vi "Get Range.vi"(11 "Exponential Fit in":refnum<class "Exponential Fit.lvclass">) -> (0 "Ymax":dbl, 1 "Ymin":dbl, 2 "Y Range":dbl, 3 "Exponential Fit out":refnum<class "Exponential Fit.lvclass">)   [LabVIEW 2013, in "Exponential Fit.lvclass"]
uses:
  Exponential Fit.lvclass
  Exponential Fit.lvclass/Exponential Fit.ctl
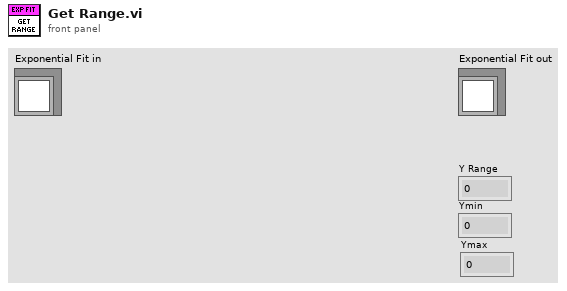
[diagram p1: front panel]
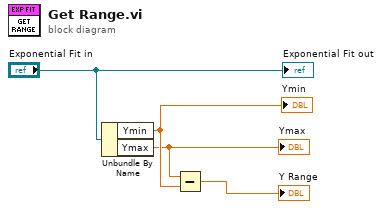
[diagram p0: block diagram]
diagram:
  n1 = Unbundle By Name("Exponential Fit in") -> ("Ymin"=w3:dbl, "Ymax"=w2:dbl)
  "Ymin" <- w3
  "Ymax" <- w2
  n2 = Subtract(x=w2, y=w3) -> (x-y=→"Y Range":dbl)
  "Exponential Fit out" <- "Exponential Fit in"
